vi "moveToPosition.vi"(0 "DMXJSAController in":refnum<class "DMXJSAController.lvclass">, 2 "target(s) (in)":T1[](array[typedef]), 5 "error in (no error)":errorcluster) -> (14 "DMXJSAController out":refnum<class "DMXJSAController.lvclass">, 17 "success?":bool, 18 "response":string, 19 "error out":errorcluster)   [LabVIEW 2020, in "classes.lvlib" / "DMXJSAController.lvclass"]
uses:
  DMXJSAController.lvclass
  C:/GEECS/Developers Version/source/Device Drivers/Newmark-NSC-A/Arcus Driver 3.0.0/ArcusUsbComm/classes/Controller/_Controller.lvclass
  movement_item.ctl
  axis.ctl
  _Controller.lvclass
  common.lvlib
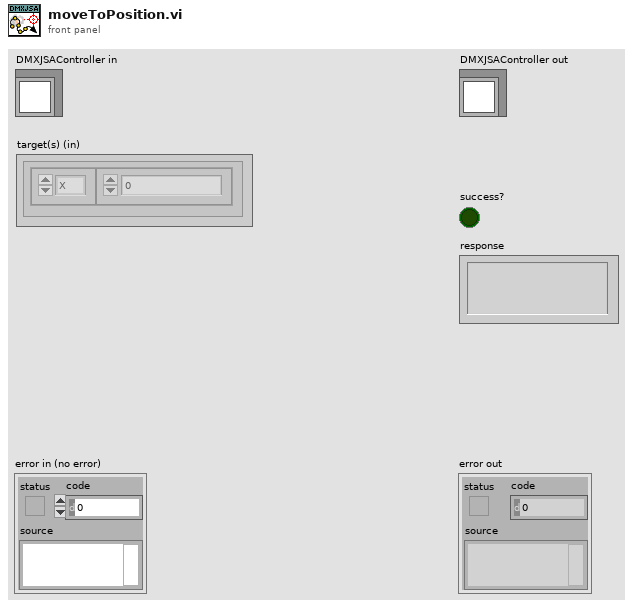
[diagram p1: front panel]
types:
  T1 = typedef "common.lvlib/movement_item.ctl" = cluster{"axis":T2, "target":i32}
  T2 = typedef "common.lvlib/axis.ctl" = enum16{"X", "Y", "Z", "U"}
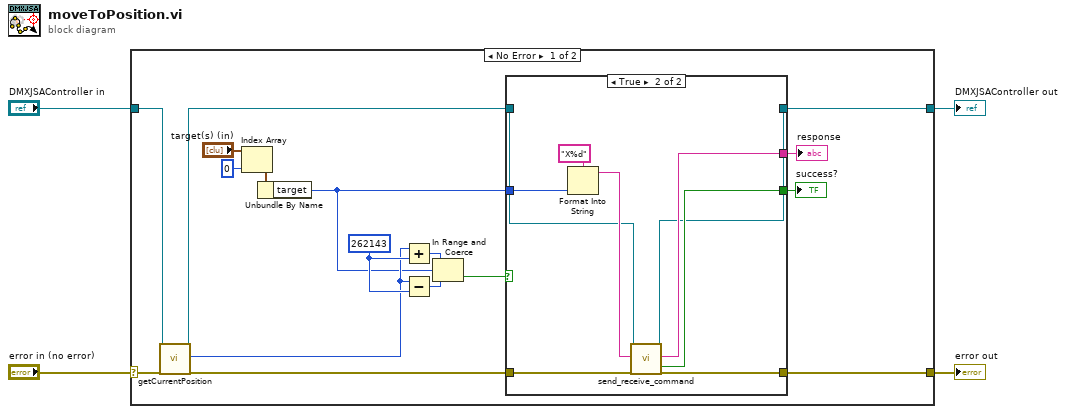
[diagram p0: block diagram]
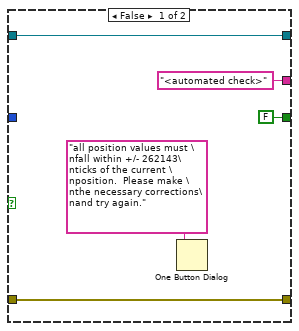
[diagram p2: hidden frame]
diagram:
  n1 = case shown="No Error" "error in (no error)" {
    selector: "error in (no error)" -> [w17 w37]
    tunnel: [w19 w37] -> w3
    tunnel: [w18 w36] -> w1
    tunnel: "DMXJSAController in" -> [w15 w36]
    frame No Error {
      w13 = 262143
      n2 = call-dynamic "getCurrentPosition.vi"("reference (in)"=w15, "error in (no error)"=w17) -> ("reference (out)"=w14:refnum<class "DMXJSAController.lvclass">, "current_position (units)"=w10:i32, "error out"=w16:errorcluster)  [unwired: 15 in]
      n3 = Index Array(array="target(s) (in)", index=0) -> (element=w6:T1)
      n4 = Unbundle By Name(w6) -> ("target"=w5:i32)
      n5 = Add(x=w10, y=w13) -> (x+y=w11:i32)
      n6 = Subtract(x=w10, y=w13) -> (x-y=w12:i32)
      n7 = In Range and Coerce(upper limit=w11, x=w5, lower limit=w12) -> (In Range?=w9:bool)  [unwired: 1 out]
      n8 = case shown="True" w9 {
        tunnel: ["<automated check>" ("response (out)") w33] -> w21
        tunnel: [FALSE ("success?") w32] -> w20
        tunnel: [w23 w31] -> w19
        tunnel: [w22 w30] -> w18
        tunnel: w16 -> [w23 w29]
        tunnel: w14 -> [w22 w28]
        tunnel: w5 -> [_ w27]
        frame False {
          n9 = One Button Dialog(message="all position values must \nfall within +/- 262143\nticks of the current \nposition.  Please make \nthe necessary corrections\nand try again.") -> ()  [unwired: 1 in, 1 out]
        }
        frame True {
          n10 = Format Into String(format string="X%d", w27) -> (resulting string=w34:string)  [unwired: 2 in, 1 out]
          n11 = call "send_receive_command.vi"("reference (in)"=w28, "ASCII Command (in)"=w34, "error in (no error)"=w29) -> ("reference (out)"=w30:refnum<class "DMXJSAController.lvclass">, "response (out)"=w33:string, "success?"=w32:bool, "error out"=w31:errorcluster)  [unwired: 12 in, 1 out]
        }
      }
      "success?" <- w20
      "response" <- w21
    }
    frame Error {
    }
  }
  "error out" <- w3
  "DMXJSAController out" <- w1
